vi "configUI.vi"() -> ()   [LabVIEW 2017, in "BuckBoost editor node.lvclass"]
doc: "All child modules share this same UI. The UI allows for the configuration of Channels, Parameters, and Error Handling."
uses:
  BuckBoost editor node.lvclass
  <vilib>/NI/Configuration Framework/Node/NodeRef.ctl
  <vilib>/NI/Configuration Framework/Node/NISE_CEF_Node.lvclass
  <vilib>/NI/AMC/Message Queue.ctl
  <vilib>/NI/AMC/Message.ctl
  <vilib>/NI/Tools/Keyed Array/KeyedArray.ctl
  <vilib>/NI/Configuration Framework/Node/UserEventRef.ctl
  <vilib>/NI/Configuration Framework/Controls/EventCluster.ctl
  <vilib>/NI/DCAF/Tag Editor Core/control module/configuration/error classification setting.ctl
  <vilib>/NI/Tag Bus Module Framework/runtime/error classification.ctl
  <vilib>/NI/Configuration Framework/Node/RefreshUIEvent.ctl
  <vilib>/NI/Configuration Framework/Node/CacheState.ctl
  <vilib>/NI/Configuration Framework/Node/StopEvent.ctl
  <vilib>/NI/Configuration Framework/Node/NodeChangeEvent.ctl
  <vilib>/NI/DCAF/Tag Editor Core/Table API/Available Tag Menu/channel action event.ctl
  <vilib>/NI/DCAF/Tag Editor Core/Table API/Available Tag Menu/dialog output action.ctl
  <vilib>/NI/Tag Bus Module Framework/channel/TBM channel.lvclass
  <vilib>/NI/Tag Bus/tag/tag descriptor.lvclass
  <vilib>/NI/DCAF/Tag Editor Core/Table API/Table Manager/Call Back Ref Type Def.ctl
  <vilib>/NI/DCAF/Tag Editor Core/Configuration Editor/Classes/Engine Parent/Engine Parent Editor Node.lvclass
  <vilib>/NI/DCAF/Tag Editor Core/Configuration Editor/Classes/Module editor node/module editor node.lvclass
  C:/Program Files (x86)/National Instruments/LabVIEW 2017/vi.lib/NI/Configuration Framework/serializable node/NISE_CEF_serializable node.lvclass
  <vilib>/rvi/Analysis/control/PID/Typedef/niFpgaPID_PIGains.ctl
  <vilib>/NI/PowerElectronicsControl/Buck-Boost/RealTime/modulationConfig.ctl
  <vilib>/NI/DCAF/Tag Editor Core/Table API/Table Manager/references.ctl
  <vilib>/NI/DCAF/Tag Editor Core/Table API/Table Manager/Menu Definition.ctl
  <vilib>/NI/DCAF/Tag Editor Core/Table API/Table Manager/Menu Options.ctl
  <vilib>/NI/DCAF/Tag Editor Core/control module/configuration/control module configuration.lvclass
  C:/Program Files (x86)/National Instruments/LabVIEW 2017/vi.lib/NI/Configuration Framework/serializable configuration/NISE_CEF_serializable configuration.lvclass
  C:/Program Files (x86)/National Instruments/LabVIEW 2017/vi.lib/NI/DCAF/Tag Editor Core/control module/editor node/control module editor.lvclass
  C:/Program Files (x86)/National Instruments/LabVIEW 2017/vi.lib/NI/DCAF/Tag Editor Core/Configuration Editor/Classes/Module editor node/module editor node.lvclass
  module/configuration/BuckBoost configuration.lvclass
  C:/Program Files (x86)/National Instruments/LabVIEW 2017/vi.lib/NI/DCAF/Tag Editor Core/control module/configuration/control module configuration.lvclass
  C:/Program Files (x86)/National Instruments/LabVIEW 2017/vi.lib/NI/Tag Bus Module Framework/module configuration/TBM module configuration.lvclass
  module/configuration/BuckBoost configuration.lvclass/BuckBoost configuration.ctl
  <vilib>/NI/DCAF/Tag Editor Core/control module/configuration/control module configuration.lvclass/control module configuration.ctl
  <vilib>/NI/Configuration Framework/serializable configuration/NISE_CEF_serializable configuration.lvclass/NISE_CEF_serializable configuration.ctl
  <vilib>/NI/Tag Bus Module Framework/channel/channel classification.ctl
  module/configuration/Read numOfInterleaves.vi
  module/configuration/Read rampRate.vi
  module/configuration/Read gains.vi
  module/configuration/Read modulationConfig.vi
  module/configuration/Write numOfInterleaves.vi
  module/configuration/Write rampRate.vi
  module/configuration/Write gains.vi
  module/configuration/Write modulationConfig.vi
  <vilib>/NI/DCAF/Tag Editor Core/control module/configuration/Write error classifications.vi
  <vilib>/NI/Tag Bus Module Framework/module configuration/TBM module configuration.lvclass
  <vilib>/NI/DCAF/Tag Editor Core/Configuration Editor/Classes/Module editor node/Read Module Configuration.vi
  <vilib>/NI/DCAF/Tag Editor Core/control module/editor node/read fixed channel configuration.vi
  <vilib>/NI/DCAF/Tag Editor Core/Configuration Editor/Classes/Module editor node/Write Module Configuration.vi
  <vilib>/Utility/LVClass/Get LV Class Name.vi
  <vilib>/NI/Configuration Framework/error generator/NISE_error generator.vi
  <vilib>/NI/Configuration Framework/serializable configuration/NISE_CEF_serializable configuration.lvclass
  <vilib>/NI/DCAF/Tag Editor Core/Table API/Listbox/Multi Column Listbox.lvclass
  <vilib>/NI/Configuration Framework/NISE_CEF_TreeControl.lvlib
  <vilib>/NI/DCAF/Tag Editor Core/Table API/Table Manager.lvlib
  <vilib>/NI/DCAF UI Toolkit/Controls/DCAF UI Elements.lvlib
  <vilib>/NI/Tools/Keyed Array/Tools_KeyedArray.lvlib
  <vilib>/NI/AMC/AMC.lvlib
  <vilib>/NI/DCAF/Tag Editor Core/Table API/Table Manager/Table Manager.lvclass
  <vilib>/NI/DCAF/Tag Editor Core/control module/editor node/control module editor.lvclass
  <vilib>/NI/Tag Bus Module Framework/runtime/TBM module execution interface.lvclass
  <vilib>/NI/PowerElectronicsControl/Buck-Boost/RealTime/BuckBoostInterface.lvlib
panel:
  in  "Enum":i32
  in  "user event out":refnum<user-event>
  in  "Top Level Tab Control":T1(tab)
  in  "rampRate":sgl
  in  "numOfInterleaves":u8
  in  "gains":T2 caption="Gains" {"proportional gain" step=0.125}
  in  "modulationConfig":T3 caption="Modulation" {"modulationRate" format="%#_6p"; "Deadband" format="%#_6p"; "SwitchingSpeed" format="%#_6p"}
  in  "Channels Listbox":i32(listbox)
  in  "mapall":bool
  in  "mapwriters":bool
  in  "Parameters Listbox":i32(listbox)
  in  "error classifications":T4[](array[typedef])
  in  "node change":T6
  in  "stop event":T7
  in  "cache state":T8
  in  "refresh UI":T9
  in  "user event":T10
  in  "main queue":T11
  in  "node ref":T12
  # "(Single-Click to Edit)"
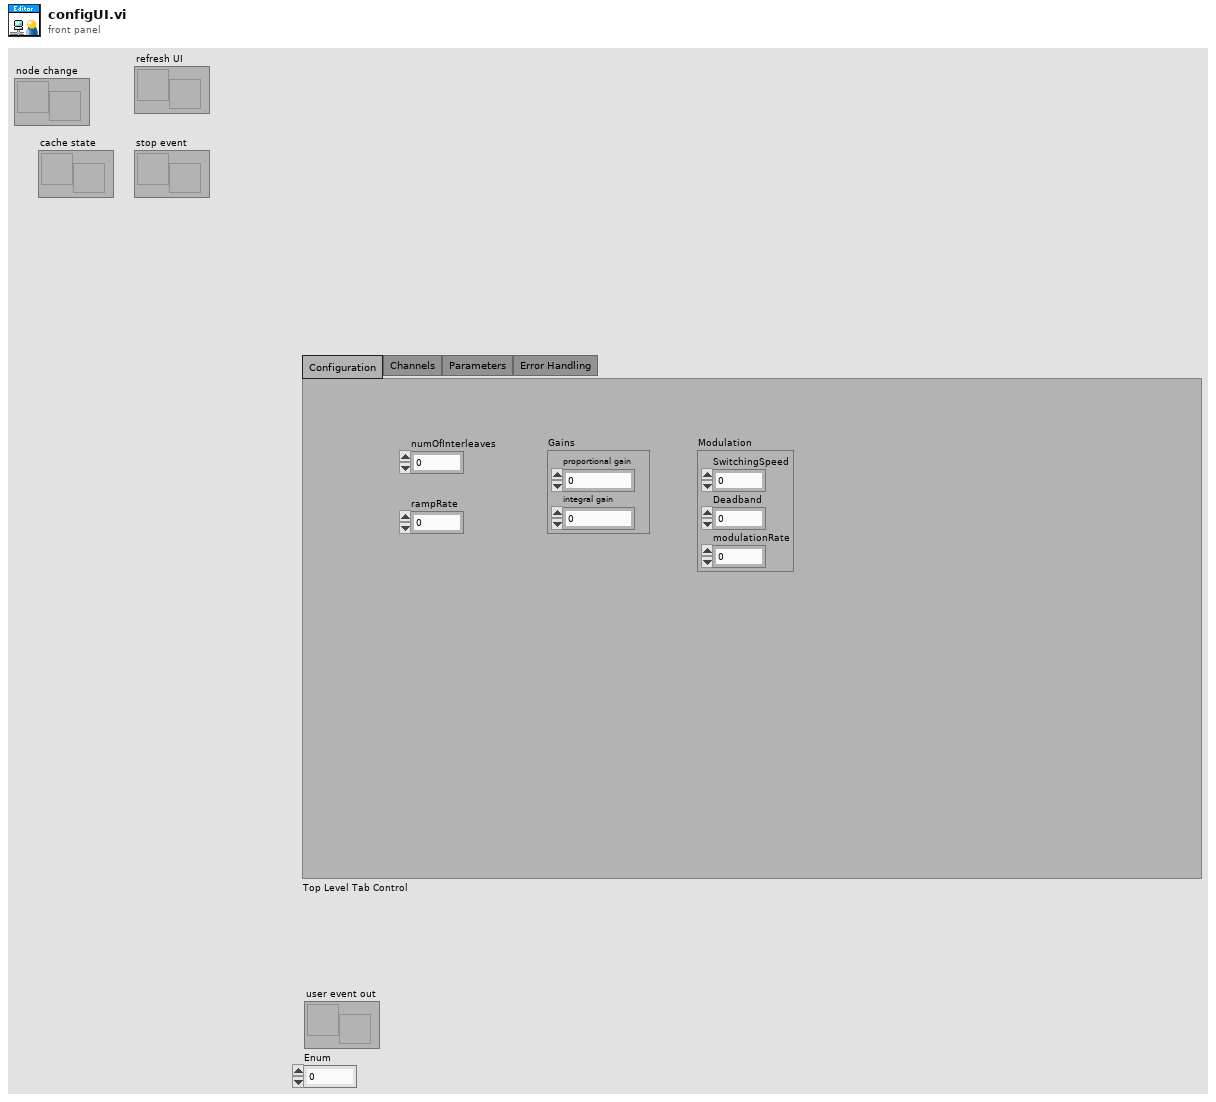
[diagram p1: front panel]
types:
  T1 = enum32{"Configuration", "Channels", "Parameters", "Error Handling"}
  T2 = typedef "niFpgaPID_PIGains.ctl" = cluster{"proportional gain":sgl, "integral gain":sgl}
  T3 = typedef "BuckBoostInterface.lvlib/modulationConfig.ctl" = cluster{"SwitchingSpeed":dbl, "Deadband":dbl, "modulationRate":dbl}
  T4 = typedef "control module configuration.lvclass/error classification setting.ctl" = cluster{"code":i32, "error classification":T5}
  T5 = typedef "TBM module execution interface.lvclass/error classification.ctl" = enum16{"unknown", "none", "trivial", "recoverable", "critical"}
  T6 = typedef "NISE_CEF_Node.lvclass/NodeChangeEvent.ctl" = refnum<user-event>
  T7 = typedef "NISE_CEF_Node.lvclass/StopEvent.ctl" = refnum<user-event>
  T8 = typedef "NISE_CEF_Node.lvclass/CacheState.ctl" = refnum<user-event>
  T9 = typedef "NISE_CEF_Node.lvclass/RefreshUIEvent.ctl" = refnum<user-event>
  T10 = typedef "NISE_CEF_Node.lvclass/UserEventRef.ctl" = refnum<user-event>
  T11 = typedef "AMC.lvlib/Message Queue.ctl" = refnum<queue>
  T12 = typedef "NISE_CEF_Node.lvclass/NodeRef.ctl" = refnum<data-value>
  T13 = typedef "Table Manager.lvlib/Table Manager.lvclass/Menu Definition.ctl" = cluster{"Menu Name":string, "Menu Options":T14}
  T14 = typedef "Table Manager.lvlib/Table Manager.lvclass/Menu Options.ctl" = enum16{"Always Show", "Show When Used", "Show When Empty"}
  T15 = typedef "Table Manager.lvlib/Table Manager.lvclass/references.ctl" = cluster{"stop event":T7, "refresh UI":T9, "cache state":T8, "node change":T6, "user event out":refnum<user-event>, "main queue":T11, "user event":T10}
  T16 = typedef "Table Manager.lvlib/Column.lvclass/Column Descriptor.ctl" = cluster{"name":string, "caption":string, "Column Type":T17, "Params":string, "AutoSizeMode":i32, "FillWeight":sgl, "MinWidth":u32, "tooltip":string, "Enum Reference":refnum<vi>, "Channel suffix":string, "Read Only":bool, "Call Back VI":T18, "DT Dependency":i32, "name dependency":i32, "data type":T19, "Custom Column":refnum<class "Column.lvclass">}
  T17 = typedef "Table Manager.lvlib/Column.lvclass/Column Type.ctl" = enum16{"String", "Mapping", "Enum", "Custom"}
  T18 = typedef "Table Manager.lvlib/Table Manager.lvclass/Call Back Ref Type Def.ctl" = refnum<vi>
  T19 = typedef "tag bus.lvlib/tag descriptor.lvclass/Data Type.ctl" = enum16{"Double", "Single", "I64", "I32", "I16", "I8", "U64", "U32", "U16", "U8", "Boolean", "String", "Array of Double", "Array of Single", "Array of I64", "Array of I32", "Array of I16", "Array of I8", "Array of U64", "Array of U32", "Array of U16", "Array of U8", "Array of Boolean", "Array of String"}
  T20 = typedef "Table Manager.lvlib/Table Manager.lvclass/object ref.ctl" = cluster{"engine":refnum<data-value>, "Node Ref":refnum<data-value>}
  T21 = typedef "Table Manager.lvlib/Table Manager.lvclass/Table Events.ctl" = cluster{"Menu Selection":refnum<user-event>}
  T22 = typedef "NISE_CEF_TreeControl.lvlib/EventCluster.ctl" = cluster{"command":string, "data":string}
  T23 = typedef "TBM channel.lvclass/channel classification.ctl" = enum16{"input data", "output data", "processing parameter", "processing result"}
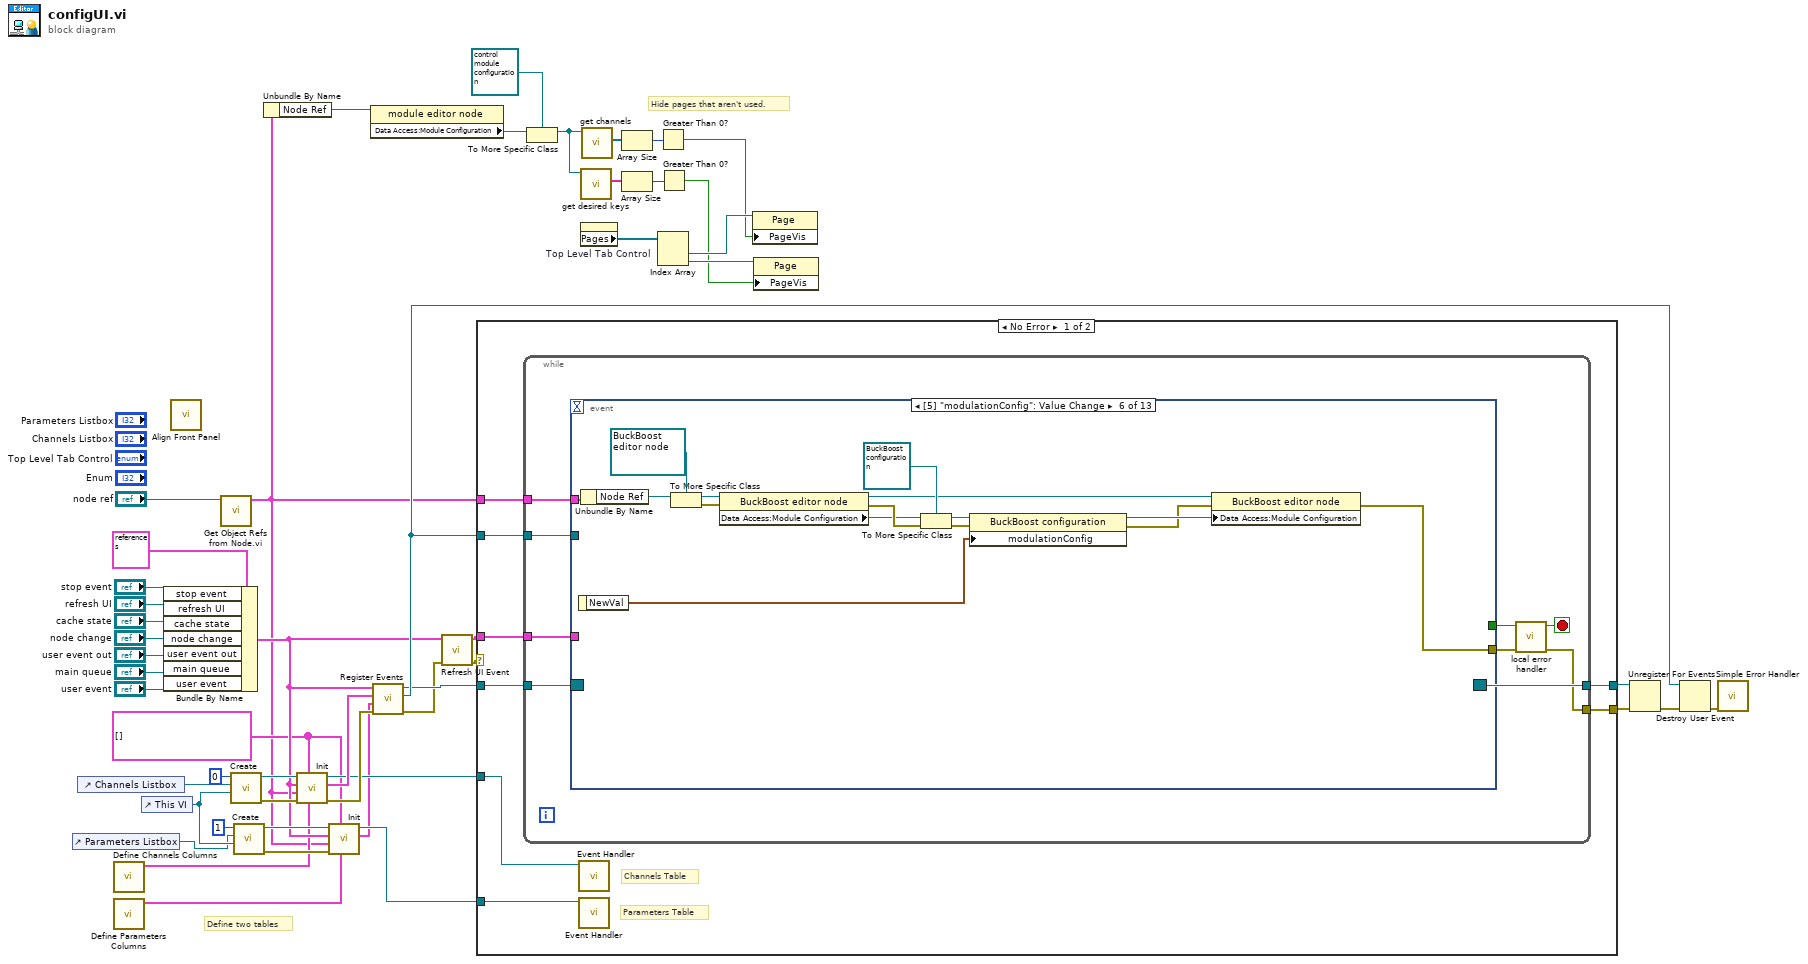
[diagram p0: block diagram]
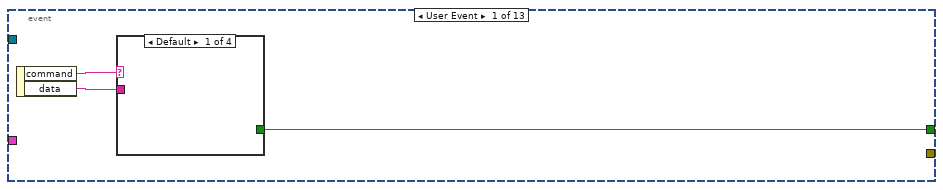
[diagram p2: hidden frame]
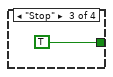
[diagram p4: hidden frame]
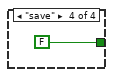
[diagram p5: hidden frame]
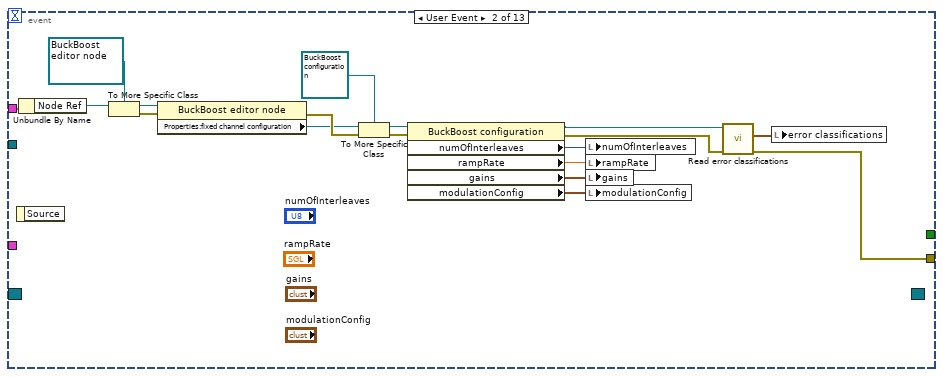
[diagram p6: hidden frame]
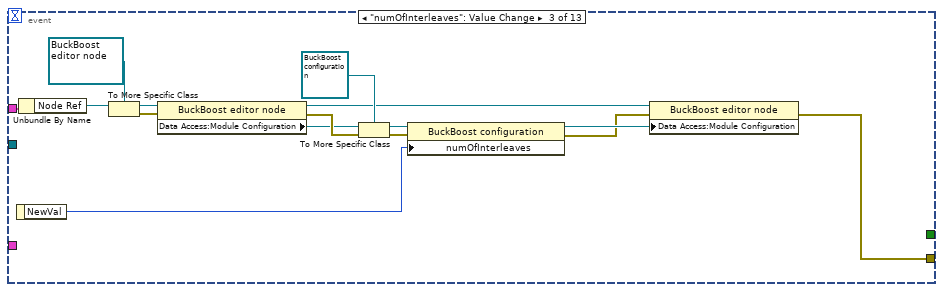
[diagram p7: hidden frame]
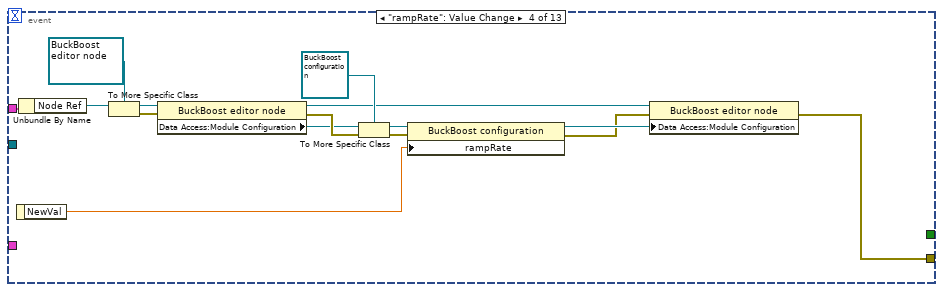
[diagram p8: hidden frame]
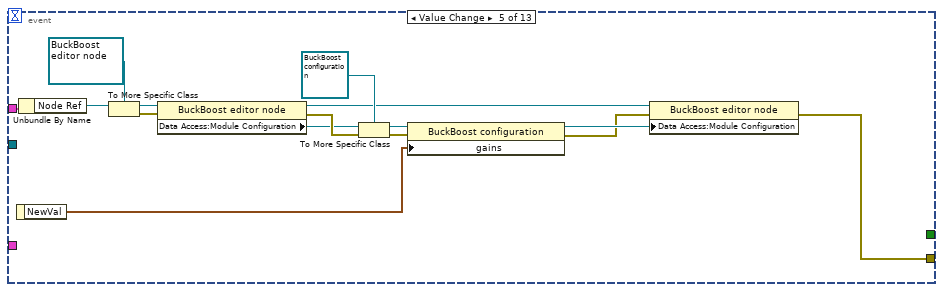
[diagram p9: hidden frame]
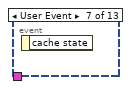
[diagram p10: hidden frame]
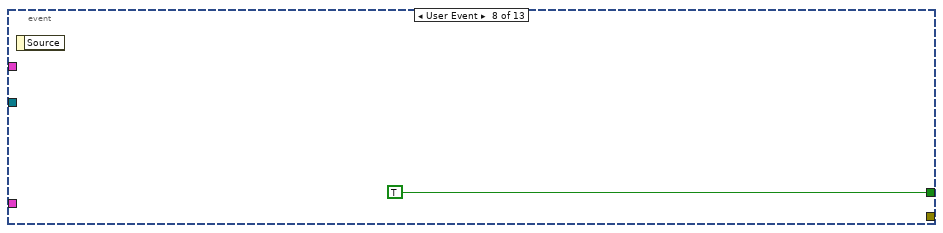
[diagram p11: hidden frame]
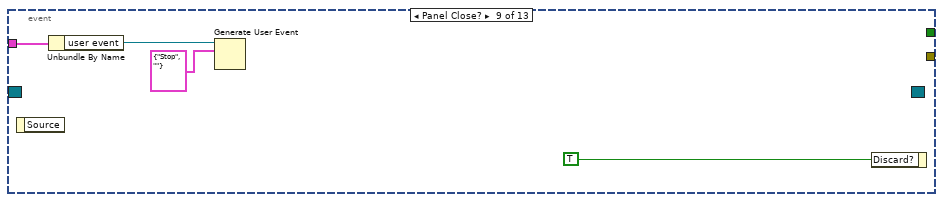
[diagram p12: hidden frame]
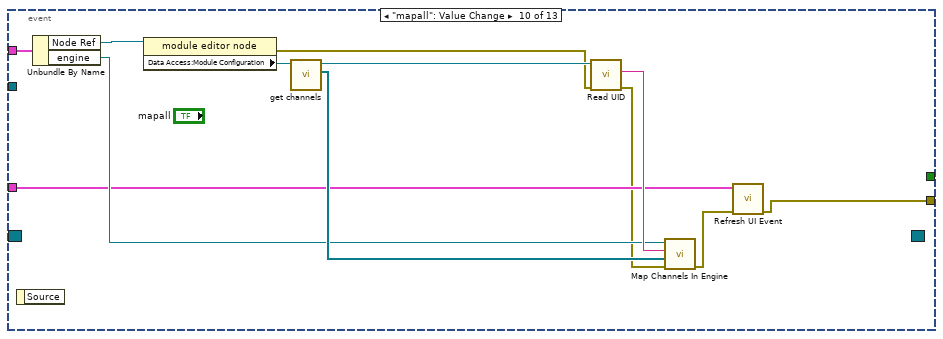
[diagram p13: hidden frame]
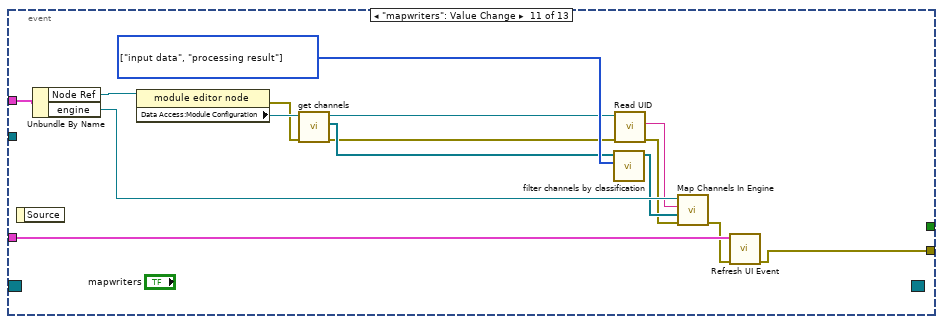
[diagram p14: hidden frame]
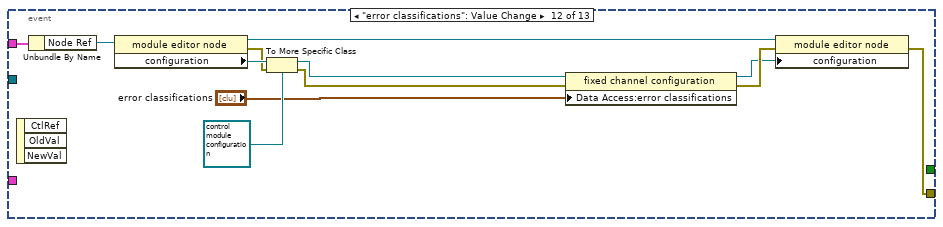
[diagram p15: hidden frame]
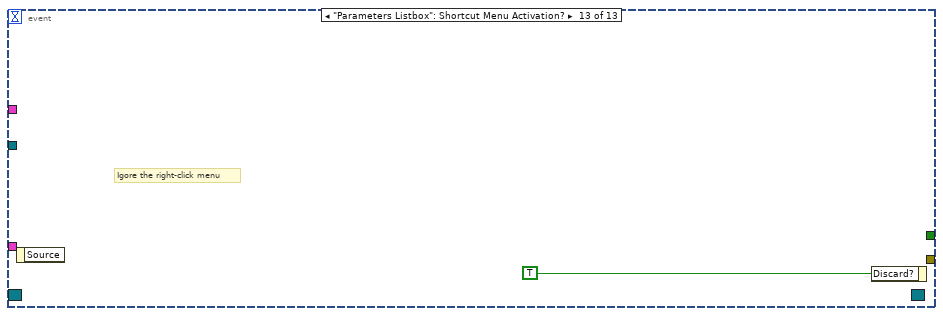
[diagram p16: hidden frame]
diagram:
  w15 = T13[] [] ("Right-Click Menu")
  # "Define two tables"
  # "Hide pages that aren't used."
  n1 = control-ref of="Parameters Listbox"() -> (w18:refnum<vi>)
  n2 = control-ref of="Channels Listbox"() -> (w26:refnum<vi>)
  n3 = call <vilib>:"Define Channels Columns.vi"() -> ("Column Descriptors"=w17:T16[])  [unwired: 11 in]
  n4 = call <vilib>:"Define Parameters Columns.vi"() -> ("Column Descriptors"=w16:T16[])  [unwired: 11 in]
  n5 = control-ref of="This VI"() -> (w22:refnum<vi>)
  n6 = Bundle By Name(cluster=T15 {"stop event"=refnum, "refresh UI"=refnum, "cache state"=refnum, "node change"=refnum, "user event out"=refnum, "main queue"=refnum, "user event"=refnum} ("Event References"), "stop event"="stop event", "refresh UI"="refresh UI", "cache state"="cache state", "node change"="node change", "user event out"="user event out", "main queue"="main queue", "user event"="user event") -> (w19:T15)
  n7 = call <vilib>:"Align Front Panel.vi"() -> ()  [unwired: 10 in, 2 out]
  n8 = call <vilib>:"Get Object Refs from Node.vi.vi"("node ref"="node ref") -> ("Node object refs"=w7:T20)  [unwired: 9 in, 1 out]
  n9 = call <vilib>:"Create.vi"("Top VI"=w22, "Listbox"=w26, "Index"=0) -> ("error out"=w29:errorcluster, "reference out"=w30:refnum<class "Multi Column Listbox.lvclass">)  [unwired: 7 in]
  n10 = call <vilib>:"Create.vi"("Top VI"=w22, "Listbox"=w18, "Index"=1) -> ("error out"=w25:errorcluster, "reference out"=w24:refnum<class "Multi Column Listbox.lvclass">)  [unwired: 7 in]
  n11 = Unbundle By Name(w7) -> ("Node Ref"=w5:refnum<data-value>)
  n12 = call-dynamic "Init.vi"("Column Descriptors"=w17, "Right-Click Menu"=w15, "error in (no error)"=w29, "Node object refs"=w7, "Event References"=w19, "Multi Column Listbox in"=w30) -> ("error out"=w28:errorcluster, "Table Events"=w40:T21, "Multi Column Listbox out"=w27:refnum<class "Multi Column Listbox.lvclass">)  [unwired: 3 in]
  n13 = call-dynamic "Init.vi"("Column Descriptors"=w16, "Right-Click Menu"=w15, "error in (no error)"=w25, "Node object refs"=w7, "Event References"=w19, "Multi Column Listbox in"=w24) -> ("Table Events"=w20:T21, "Multi Column Listbox out"=w21:refnum<class "Multi Column Listbox.lvclass">)  [unwired: 3 in, 1 out]
  n14 = property class="module editor node"(reference=w5) -> ("Data Access:Module Configuration"=w6:refnum<class "TBM module configuration.lvclass">)  [unwired: 1 in, 2 out]
  n15 = call <vilib>:"Register Events.vi"("error in (no error)"=w28, "Parameters Table Events"=w20, "Channels Table Events"=w40, "Event References"=w19) -> ("error out"=w33:errorcluster, "Channel Action"=w39:refnum<user-event>, "Event Registration Refnum"=w38:refnum<event-registration>)  [unwired: 5 in]
  n16 = call <vilib>:"Refresh UI Event.vi"("error in (no error)"=w33, "Event References"=w19) -> ("error out"=w34:errorcluster, "Event References out"=w32:T15)  [unwired: 8 in]
  n17 = case shown="No Error" w34 {
    selector: w34 -> [_ w196]
    tunnel: w38 -> [w58 w195]
    tunnel: [w57 w195] -> w50
    tunnel: [w55 w196] -> w49
    tunnel: w39 -> [w56 _]
    tunnel: w7 -> [w54 _]
    tunnel: w32 -> [w53 _]
    tunnel: w27 -> [w52 _]
    tunnel: w21 -> [w51 _]
    frame No Error {
      # "Parameters Table"
      # "Channels Table"
      n18 = while {
        tunnel: w58 -> [w67]
        tunnel: [w66] -> w57
        tunnel: w56 -> [w65]
        tunnel: [w61] -> w55
        tunnel: w54 -> [w60]
        tunnel: w53 -> [w59]
        stop <- w63 stop-if-true
        n19 = event shown="[5] \"modulationConfig\": Value Change" {
          selector: w67 -> [_ _ _ _ _ _ _ _ _ _ _ _ _]
          dyn-events: [_ _ _ _ _ _ _ _ _ _ _ _ _] -> w66
          timeout: _ -> [_ _ _ _ _ _ _ _ _ _ _ _ _]
          tunnel: [w70 _ _ _ _ _ _ TRUE _ _ _ _ _] -> w64
          tunnel: [_ w88 w91 w106 w121 w136 _ _ _ w161 w177 w193 _] -> w62
          tunnel: w65 -> [_ _ _ _ _ _ _ _ _ _ _ _ _]
          tunnel: w60 -> [_ w90 w105 w120 w135 w150 _ _ _ w165 w178 w192 _]
          tunnel: w59 -> [_ _ _ _ _ _ _ _ w153 w160 w176 _ _]
          event User Event {
            n20 = event-data() -> ("command"=w69:string, "data"=w68:string)  [unwired: 1 in]
            n21 = case shown="Default" w69 {
              tunnel: [_ _ TRUE FALSE] -> w70
              tunnel: w68 -> [_ _ _ _]
              frame Default {
              }
              frame "Refresh" {
              }
              frame "Stop" {
              }
              frame "save" {
              }
            }
          }
          event User Event {
            n22 = event-data() -> ()  [unwired: 1 in, 1 out]
            n23 = Unbundle By Name(w90) -> ("Node Ref"=w89:refnum<data-value>)
            n24 = To More Specific Class(target class=refnum<data-value> refnum ("data value reference"), reference=w89) -> (specific class reference=w87:refnum<data-value>, error out=w83:errorcluster)  [unwired: 1 in]
            n25 = property class="BuckBoost editor node"(reference=w87, error in=w83) -> (error out=w84:errorcluster, "Properties:fixed channel configuration"=w82:refnum<class "control module configuration.lvclass">)  [unwired: 1 out]
            n26 = To More Specific Class(target class=refnum<class "BuckBoost configuration.lvclass"> refnum ("BuckBoost configuration"), reference=w82, error in=w84) -> (specific class reference=w80:refnum<class "BuckBoost configuration.lvclass">, error out=w79:errorcluster)
            n27 = property class="BuckBoost configuration"(reference=w80, error in=w79) -> (reference out=w78:refnum<class "BuckBoost configuration.lvclass">, error out=w77:errorcluster, "numOfInterleaves"=w73:u8, "rampRate"=w74:sgl, "gains"=w75:T2, "modulationConfig"=w76:T3)
            n28 = local write "numOfInterleaves"(w73) -> ()
            n29 = local write "rampRate"(w74) -> ()
            n30 = local write "gains"(w75) -> ()
            n31 = local write "modulationConfig"(w76) -> ()
            n32 = call <vilib>:"Read error classifications.vi"("error in"=w77, "control module configuration in"=w78) -> ("error out"=w88:errorcluster, "error classifications"=w86:T4[])  [unwired: 7 in, 1 out]
            n33 = local write "error classifications"(w86) -> ()
          }
          event "numOfInterleaves": Value Change {
            n34 = event-data() -> ("NewVal"=w95:u8)  [unwired: 1 in]
            n35 = Unbundle By Name(w105) -> ("Node Ref"=w104:refnum<data-value>)
            n36 = To More Specific Class(target class=refnum<data-value> refnum ("data value reference"), reference=w104) -> (specific class reference=w103:refnum<data-value>, error out=w100:errorcluster)  [unwired: 1 in]
            n37 = property class="BuckBoost editor node"(reference=w103, error in=w100) -> (reference out=w94:refnum<data-value>, error out=w101:errorcluster, "Data Access:Module Configuration"=w99:refnum<class "TBM module configuration.lvclass">)
            n38 = To More Specific Class(target class=refnum<class "BuckBoost configuration.lvclass"> refnum ("BuckBoost configuration"), reference=w99, error in=w101) -> (specific class reference=w97:refnum<class "BuckBoost configuration.lvclass">, error out=w96:errorcluster)
            n39 = property class="BuckBoost configuration"(reference=w97, error in=w96, "numOfInterleaves"=w95) -> (reference out=w93:refnum<class "BuckBoost configuration.lvclass">, error out=w92:errorcluster)
            n40 = property class="BuckBoost editor node"(reference=w94, error in=w92, "Data Access:Module Configuration"=w93) -> (error out=w91:errorcluster)  [unwired: 1 out]
          }
          event "rampRate": Value Change {
            n41 = event-data() -> ("NewVal"=w110:sgl)  [unwired: 1 in]
            n42 = Unbundle By Name(w120) -> ("Node Ref"=w119:refnum<data-value>)
            n43 = To More Specific Class(target class=refnum<data-value> refnum ("data value reference"), reference=w119) -> (specific class reference=w118:refnum<data-value>, error out=w115:errorcluster)  [unwired: 1 in]
            n44 = property class="BuckBoost editor node"(reference=w118, error in=w115) -> (reference out=w109:refnum<data-value>, error out=w116:errorcluster, "Data Access:Module Configuration"=w114:refnum<class "TBM module configuration.lvclass">)
            n45 = To More Specific Class(target class=refnum<class "BuckBoost configuration.lvclass"> refnum ("BuckBoost configuration"), reference=w114, error in=w116) -> (specific class reference=w112:refnum<class "BuckBoost configuration.lvclass">, error out=w111:errorcluster)
            n46 = property class="BuckBoost configuration"(reference=w112, error in=w111, "rampRate"=w110) -> (reference out=w108:refnum<class "BuckBoost configuration.lvclass">, error out=w107:errorcluster)
            n47 = property class="BuckBoost editor node"(reference=w109, error in=w107, "Data Access:Module Configuration"=w108) -> (error out=w106:errorcluster)  [unwired: 1 out]
          }
          event Value Change {
            n48 = event-data() -> ("NewVal"=w125:T2)  [unwired: 1 in]
            n49 = Unbundle By Name(w135) -> ("Node Ref"=w134:refnum<data-value>)
            n50 = To More Specific Class(target class=refnum<data-value> refnum ("data value reference"), reference=w134) -> (specific class reference=w133:refnum<data-value>, error out=w130:errorcluster)  [unwired: 1 in]
            n51 = property class="BuckBoost editor node"(reference=w133, error in=w130) -> (reference out=w124:refnum<data-value>, error out=w131:errorcluster, "Data Access:Module Configuration"=w129:refnum<class "TBM module configuration.lvclass">)
            n52 = To More Specific Class(target class=refnum<class "BuckBoost configuration.lvclass"> refnum ("BuckBoost configuration"), reference=w129, error in=w131) -> (specific class reference=w127:refnum<class "BuckBoost configuration.lvclass">, error out=w126:errorcluster)
            n53 = property class="BuckBoost configuration"(reference=w127, error in=w126, "gains"=w125) -> (reference out=w123:refnum<class "BuckBoost configuration.lvclass">, error out=w122:errorcluster)
            n54 = property class="BuckBoost editor node"(reference=w124, error in=w122, "Data Access:Module Configuration"=w123) -> (error out=w121:errorcluster)  [unwired: 1 out]
          }
          event Value Change {
            n55 = event-data() -> ("NewVal"=w140:T3)  [unwired: 1 in]
            n56 = Unbundle By Name(w150) -> ("Node Ref"=w149:refnum<data-value>)
            n57 = To More Specific Class(target class=refnum<data-value> refnum ("data value reference"), reference=w149) -> (specific class reference=w148:refnum<data-value>, error out=w145:errorcluster)  [unwired: 1 in]
            n58 = property class="BuckBoost editor node"(reference=w148, error in=w145) -> (reference out=w139:refnum<data-value>, error out=w146:errorcluster, "Data Access:Module Configuration"=w144:refnum<class "TBM module configuration.lvclass">)
            n59 = To More Specific Class(target class=refnum<class "BuckBoost configuration.lvclass"> refnum ("BuckBoost configuration"), reference=w144, error in=w146) -> (specific class reference=w142:refnum<class "BuckBoost configuration.lvclass">, error out=w141:errorcluster)
            n60 = property class="BuckBoost configuration"(reference=w142, error in=w141, "modulationConfig"=w140) -> (reference out=w138:refnum<class "BuckBoost configuration.lvclass">, error out=w137:errorcluster)
            n61 = property class="BuckBoost editor node"(reference=w139, error in=w137, "Data Access:Module Configuration"=w138) -> (error out=w136:errorcluster)  [unwired: 1 out]
          }
          event User Event {
            n62 = event-data() -> ()  [unwired: 1 in, 1 out]
          }
          event User Event {
            n63 = event-data() -> ()  [unwired: 1 in, 1 out]
          }
          event Panel Close? {
            n64 = event-data() -> ()  [unwired: 1 in, 1 out]
            n65 = Unbundle By Name(w153) -> ("user event"=w152:T10)
            n66 = Generate User Event(user event=w152, event data cluster=T22 {"command"="Stop", "data"=""} ("event data")) -> ()  [unwired: 2 in, 2 out]
            n67 = event-data("Discard?"=TRUE) -> ()  [unwired: 1 in, 1 out]
          }
          event "mapall": Value Change {
            n68 = event-data() -> ()  [unwired: 1 in, 1 out]
            n69 = Unbundle By Name(w165) -> ("Node Ref"=w164:refnum<data-value>, "engine"=w163:refnum<data-value>)
            n70 = property class="module editor node"(reference=w164) -> (error out=w157:errorcluster, "Data Access:Module Configuration"=w159:refnum<class "TBM module configuration.lvclass">)  [unwired: 1 in, 1 out]
            n71 = call-dynamic "get channels.vi"("module configuration in"=w159) -> ("channels"=w167:refnum<class "TBM channel.lvclass">[], "module configuration out"=w158:refnum<class "TBM module configuration.lvclass">)  [unwired: 9 in]
            n72 = call <vilib>:"Read UID.vi"("error in"=w157, "configuration in"=w158) -> ("error out"=w156:errorcluster, "instance id"=w166:string)  [unwired: 7 in, 1 out]
            n73 = call <vilib>:"Map Channels In Engine.vi"("error in (no error)"=w156, "channels"=w167, "instance id"=w166, "Engine DVR"=w163) -> ("error out"=w162:errorcluster)  [unwired: 7 in]
            n74 = call <vilib>:"Refresh UI Event.vi"("error in (no error)"=w162, "Event References"=w160) -> ("error out"=w161:errorcluster)  [unwired: 8 in, 1 out]
          }
          event "mapwriters": Value Change {
            w181 = T23[] [enum."input data", enum."processing result"] items=["input data", "output data", "processing parameter", "processing result"] ("allowed classifications")
            n75 = event-data() -> ()  [unwired: 1 in, 1 out]
            n76 = Unbundle By Name(w178) -> ("Node Ref"=w179:refnum<data-value>, "engine"=w175:refnum<data-value>)
            n77 = property class="module editor node"(reference=w179) -> (error out=w168:errorcluster, "Data Access:Module Configuration"=w170:refnum<class "TBM module configuration.lvclass">)  [unwired: 1 in, 1 out]
            n78 = call-dynamic "get channels.vi"("module configuration in"=w170) -> ("channels"=w180:refnum<class "TBM channel.lvclass">[], "module configuration out"=w169:refnum<class "TBM module configuration.lvclass">)  [unwired: 9 in]
            n79 = call <vilib>:"filter channels by classification.vi"("allowed classifications"=w181, "channels in"=w180) -> ("channels out"=w173:refnum<class "TBM channel.lvclass">[])  [unwired: 9 in]
            n80 = call <vilib>:"Read UID.vi"("error in"=w168, "configuration in"=w169) -> ("error out"=w172:errorcluster, "instance id"=w174:string)  [unwired: 7 in, 1 out]
            n81 = call <vilib>:"Map Channels In Engine.vi"("error in (no error)"=w172, "channels"=w173, "instance id"=w174, "Engine DVR"=w175) -> ("error out"=w171:errorcluster)  [unwired: 7 in]
            n82 = call <vilib>:"Refresh UI Event.vi"("error in (no error)"=w171, "Event References"=w176) -> ("error out"=w177:errorcluster)  [unwired: 8 in, 1 out]
          }
          event "error classifications": Value Change {
            n83 = event-data() -> ()  [unwired: 1 in, 3 out]
            n84 = Unbundle By Name(w192) -> ("Node Ref"=w187:refnum<data-value>)
            n85 = property class="module editor node"(reference=w187) -> (reference out=w191:refnum<data-value>, error out=w183:errorcluster, "configuration"=w186:refnum<class "NISE_CEF_serializable configuration.lvclass">)  [unwired: 1 in]
            n86 = To More Specific Class(target class=refnum<class "control module configuration.lvclass"> refnum ("fixed channel configuration"), reference=w186, error in=w183) -> (specific class reference=w188:refnum<class "control module configuration.lvclass">, error out=w182:errorcluster)
            n87 = property class="fixed channel configuration"(reference=w188, error in=w182, "Data Access:error classifications"="error classifications") -> (reference out=w189:refnum<class "control module configuration.lvclass">, error out=w190:errorcluster)
            n88 = property class="module editor node"(reference=w191, error in=w190, "configuration"=w189) -> (error out=w193:errorcluster)  [unwired: 1 out]
          }
          event "Parameters Listbox": Shortcut Menu Activation? {
            # "Igore the right-click menu"
            n89 = event-data() -> ()  [unwired: 1 in, 1 out]
            n90 = event-data("Discard?"=TRUE) -> ()  [unwired: 1 in, 1 out]
          }
        }
        n91 = call <vilib>:"local error handler.vi"("error in (no error)"=w62, "Stop in"=w64) -> ("error out"=w61:errorcluster, "Stop out"=w63:bool)  [unwired: 8 in]
      }
      n92 = call-dynamic "Event Handler.vi"("Listbox in"=w52) -> ()  [unwired: 9 in, 2 out]
      n93 = call-dynamic "Event Handler.vi"("Listbox in"=w51) -> ()  [unwired: 9 in, 2 out]
    }
    frame Error {
    }
  }
  n94 = To More Specific Class(target class=refnum<class "control module configuration.lvclass"> refnum ("fixed channel configuration"), reference=w6) -> (specific class reference=w3:refnum<class "control module configuration.lvclass">)  [unwired: 1 in, 1 out]
  n95 = call-dynamic "get desired keys.vi"("fixed channel configuration in"=w3) -> ("desired keys"=w11:string[])  [unwired: 8 in, 2 out]
  n96 = property on="Top Level Tab Control" class="TabCtl (strict)"() -> ("Pages"=w8:refnum<vi>[])  [unwired: 2 in, 2 out]
  n97 = call-dynamic "get channels.vi"("fixed channel configuration in"=w3) -> ("channels"=w14:refnum<class "TBM channel.lvclass">[])  [unwired: 9 in, 1 out]
  n98 = Array Size(array=w14) -> (size(s)=w13:i32)
  n99 = Array Size(array=w11) -> (size(s)=w12:i32)
  n100 = Greater Than 0?(x=w13) -> (x > 0?=w2:bool)
  n101 = Index Array(array=w8) -> (element #1=w9:refnum<vi>, element #2=w10:refnum<vi>)  [unwired: 2 in]
  n102 = Greater Than 0?(x=w12) -> (x > 0?=w1:bool)
  n103 = property class="Page"(reference=w9, "PageVis"=w2) -> ()  [unwired: 1 in, 2 out]
  n104 = property class="Page"(reference=w10, "PageVis"=w1) -> ()  [unwired: 1 in, 2 out]
  n105 = Unregister For Events(event registration refnum=w50, error in=w49) -> (error out=w48:errorcluster)
  n106 = Destroy User Event(user event=w39, error in=w48) -> (error out=w47:errorcluster)
  n107 = call <vilib>:"Simple Error Handler.vi"("error in (no error)"=w47) -> ()  [unwired: 4 in, 5 out]
